vi "Read_Loop.vi"(8 "Status/Errors in":refnum<vi>, 9 "Read bytes parameters in":T1 {"Read bytes"."Max bytes read" format="%#.0f"}, 10 "Timer parameters":refnum<vi>, 11 "Devices":T4) -> (0 "Status/Errors out":refnum<vi>, 1 "Read bytes parameters out":T1 {"Read bytes"."Max bytes read" format="%#.0f"}, 2 "Slave bytes":u8[](array[numeric]), 3 "Master bytes":u8[](array[numeric]), 4 "# Master bytes":u32, 6 "# Slave bytes":u32)   [LabVIEW 2013]
uses:
  Controls/Read_Bytes_Parameters.ctl
  Controls/Stop_Loop.ctl
  Controls/Read_Bytes.ctl
  Controls/Devices.ctl
  Controls/Timer_Elements.ctl
  Controls/Get_Set_Timer_Options.ctl
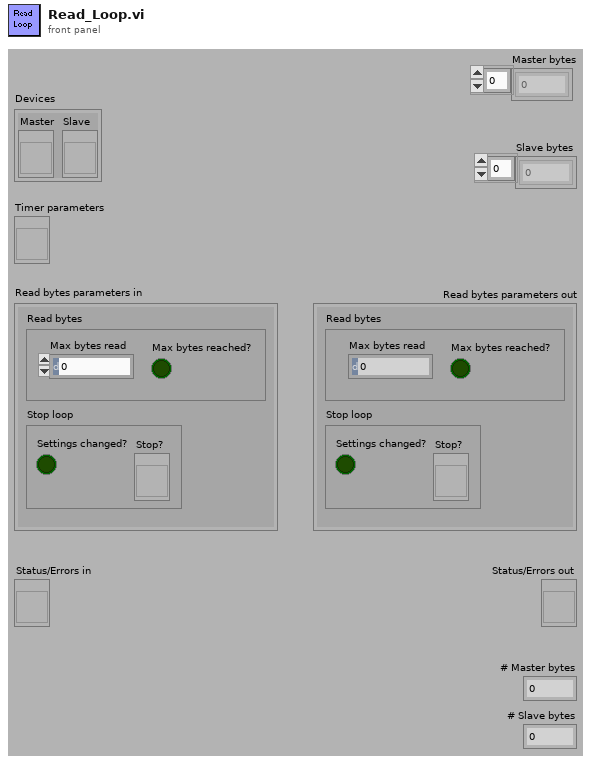
[diagram p1: front panel]
types:
  T1 = typedef "Read_Bytes_Parameters.ctl" = cluster{"Stop loop":T2, "Read bytes":T3}
  T2 = typedef "Stop_Loop.ctl" = cluster{"Settings changed?":bool, "Stop?":refnum<vi>}
  T3 = typedef "Read_Bytes.ctl" = cluster{"Max bytes read":u32, "Max bytes reached?":bool}
  T4 = typedef "Devices.ctl" = cluster{"Master":refnum<vi>, "Slave":refnum<vi>}
  T5 = typedef "Semaphore RefNum" = refnum<k1>
  T6 = typedef "Get_Set_Timer_Options.ctl" = enum16{"Get", "Get cluster", "Set", "Set to current time"}
  T7 = typedef "Timer_Elements.ctl" = enum16{"Default", "Current time", "Time screen updated", "Time controls locked", "Time last device check", "Time last data MAS", "Time last data SLV", "Time bad status MAS", "Time bad status SLV", "Time clock error updated", "Time delay screen update", "Time delay controls", "Time delay device check", "Time until MAS status bad", "Time until SLV status bad", "Time until MAS connection bad", "Time until SLV connection bad", "Time delay clock error update"}
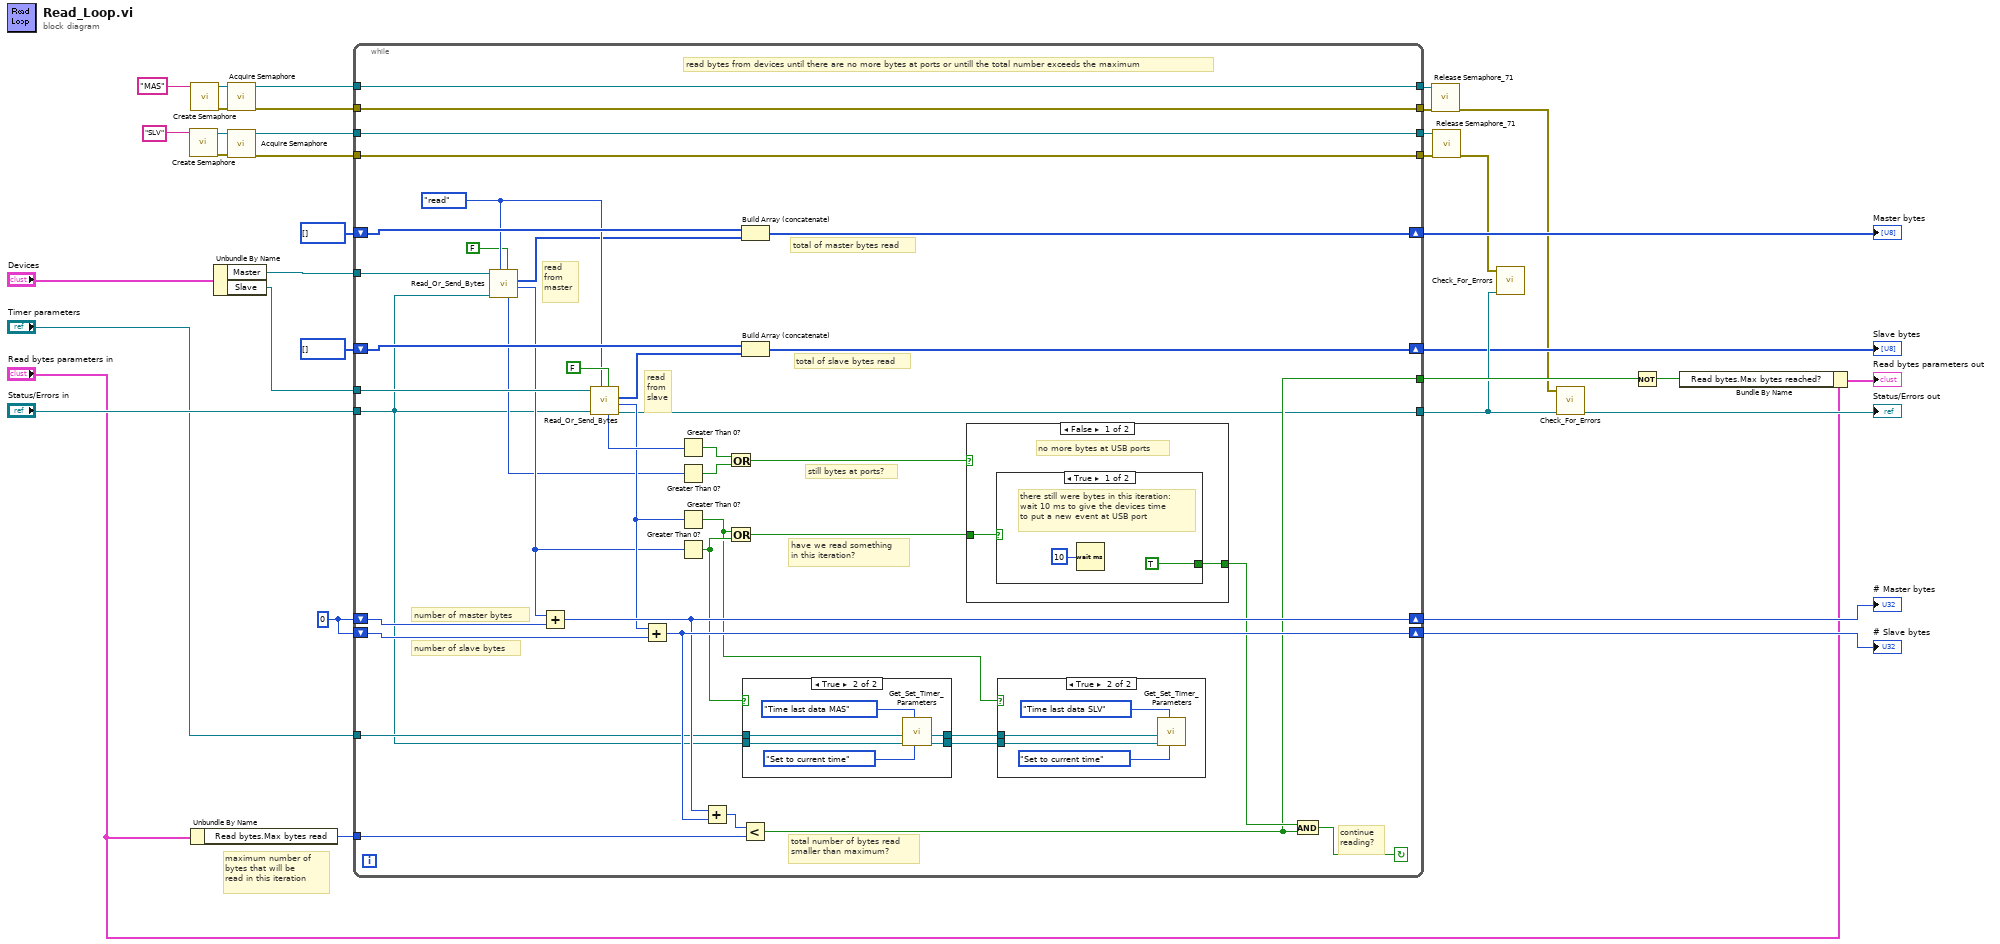
[diagram p0: block diagram]
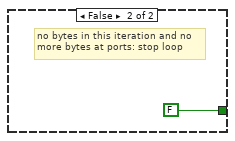
[diagram p4: hidden frame]
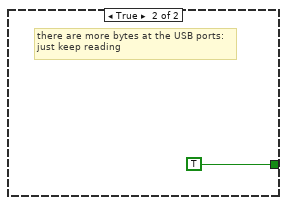
[diagram p5: hidden frame]
diagram:
  w33 = u32 0
  # "maximum number of\nbytes that will be\nread in this iteration"
  n1 = call <vilib>:"Create Semaphore.vi"("name (unnamed)"="SLV") -> ("error out"=w11:errorcluster, "semaphore"=w12:T5)  [unwired: 2 in, 3 out]
  n2 = call <vilib>:"Create Semaphore.vi"("name (unnamed)"="MAS") -> ("error out"=w7:errorcluster, "semaphore"=w8:T5)  [unwired: 2 in, 3 out]
  n3 = Unbundle By Name("Read bytes parameters in") -> ("Read bytes.Max bytes read"=w13:u32)
  n4 = Unbundle By Name("Devices") -> ("Master"=w35:refnum<vi>, "Slave"=w34:refnum<vi>)
  n5 = call <vilib>:"Acquire Semaphore.vi"("error in (no error)"=w7, "semaphore"=w8) -> ("error out"=w24:errorcluster, "semaphore out"=w25:T5)  [unwired: 1 in, 3 out]
  n6 = call <vilib>:"Acquire Semaphore.vi"("error in (no error)"=w11, "semaphore"=w12) -> ("error out"=w21:errorcluster, "semaphore out"=w22:T5)  [unwired: 1 in, 3 out]
  n7 = while {
    tunnel: "Status/Errors in" -> [w36]
    shift-right: [w69] -> w30
    shift-left: w33 -> [w72]
    tunnel: w13 -> [w74]
    shift-right: [w56] -> w17
    shift-left: u8[] [] -> [w57]
    shift-right: [w55] -> w16
    shift-left: u8[] [] -> [w54]
    shift-right: [w70] -> w29
    shift-left: w33 -> [w71]
    tunnel: w35 -> [w42]
    tunnel: w34 -> [w48]
    tunnel: [w43] -> w20
    tunnel: [w62] -> w28
    tunnel: w25 -> [w60]
    tunnel: w24 -> [w61]
    tunnel: [w61] -> w5
    tunnel: [w60] -> w4
    tunnel: w22 -> [w58]
    tunnel: w21 -> [w59]
    tunnel: [w59] -> w2
    tunnel: [w58] -> w1
    tunnel: "Timer parameters" -> [w53]
    stop <- w73 continue-if-true
    w41 = enum8{"read", "write"}."read" ("Read or write?")
    # "have we read something\nin this iteration?"
    # "number of slave bytes"
    # "number of master bytes"
    # "read\nfrom\nmaster"
    # "read\nfrom\nslave"
    # "read bytes from devices until there are no more bytes at ports or untill the total number exceeds the maximum"
    # "total of slave bytes read"
    # "total of master bytes read"
    # "continue\nreading?"
    # "total number of bytes read\nsmaller than maximum?"
    # "still bytes at ports?"
    n8 = call "Read_Or_Send_Bytes.vi"("Aquire semaphore? (t)"=FALSE, "Read or write?"=w41, "Status/Errors in"=w36, "Device in"=w42) -> ("Return count"=w38:u32, "Read buffer"=w39:u8[], "Bytes at Port"=w37:u32)  [unwired: 1 in, 4 out]
    n9 = Add(x=w38, y=w72) -> (x+y=w69:u32)
    n10 = call "Read_Or_Send_Bytes.vi"("Aquire semaphore? (t)"=FALSE, "Read or write?"=w41, "Status/Errors in"=w36, "Device in"=w48) -> ("Status/Errors out"=w43:refnum<vi>, "Return count"=w44:u32, "Read buffer"=w45:u8[], "Bytes at Port"=w46:u32)  [unwired: 1 in, 3 out]
    n11 = Add(x=w44, y=w71) -> (x+y=w70:u32)
    n12 = Greater Than 0?(x=w46) -> (x > 0?=w66:bool)
    n13 = Greater Than 0?(x=w37) -> (x > 0?=w65:bool)
    n14 = Greater Than 0?(x=w44) -> (x > 0?=w49:bool)
    n15 = Greater Than 0?(x=w38) -> (x > 0?=w50:bool)
    n16 = Add(x=w69, y=w70) -> (x+y=w68:u32)
    n17 = Or(x=w66, y=w65) -> (x .or. y?=w64:bool)
    n18 = Or(x=w49, y=w50) -> (x .or. y?=w63:bool)
    n19 = Less?(x=w68, y=w74) -> (x < y?=w62:bool)
    n20 = Build Array (concatenate)(w57, w39) -> (w56:u8[])
    n21 = Build Array (concatenate)(w54, w45) -> (w55:u8[])
    n22 = case shown="True" w50 {
      tunnel: w36 -> [w79 w84]
      tunnel: w53 -> [w80 w83]
      tunnel: [w80 w82] -> w52
      tunnel: [w79 w81] -> w51
      frame False {
      }
      frame True {
        n23 = call "Get_Set_Timer_Parameters.vi"("Get/Set"=Get_Set_Timer_Options."Set to current time", "Element"=Timer_Elements."Time last data MAS", "Status/Errors in"=w84, "Timer parameters in"=w83) -> ("Status/Errors out"=w81:refnum<vi>, "Timer parameters out"=w82:refnum<vi>)  [unwired: 2 in, 4 out]
      }
    }
    n24 = case shown="False" w64 {
      tunnel: w63 -> [w88 _]
      tunnel: [w87 TRUE] -> w67
      frame False {
        # "no more bytes at USB ports"
        n25 = case shown="True" w88 {
          tunnel: [TRUE FALSE] -> w87
          frame True {
            # "there still were bytes in this iteration:\nwait 10 ms to give the devices time\nto put a new event at USB port"
            n26 = Wait (ms)(milliseconds to wait=u32 10) -> ()  [unwired: 1 out]
          }
          frame False {
            # "no bytes in this iteration and no\nmore bytes at ports: stop loop"
          }
        }
      }
      frame True {
        # "there are more bytes at the USB ports:\njust keep reading"
      }
    }
    n27 = case shown="True" w49 {
      tunnel: w51 -> [_ w76]
      tunnel: w52 -> [_ w75]
      frame False {
      }
      frame True {
        n28 = call "Get_Set_Timer_Parameters.vi"("Get/Set"=Get_Set_Timer_Options."Set to current time", "Element"=Timer_Elements."Time last data SLV", "Status/Errors in"=w76, "Timer parameters in"=w75) -> ()  [unwired: 2 in, 6 out]
      }
    }
    n29 = And(x=w67, y=w62) -> (x .and. y?=w73:bool)
  }
  "# Master bytes" <- w30
  "# Slave bytes" <- w29
  "Master bytes" <- w17
  "Slave bytes" <- w16
  n30 = call <vilib>:"Release Semaphore_71.vi"("error in (no error)"=w5, "semaphore"=w4) -> ("error out"=w6:errorcluster)  [unwired: 5 out]
  n31 = call <vilib>:"Release Semaphore_71.vi"("error in (no error)"=w2, "semaphore"=w1) -> ("error out"=w3:errorcluster)  [unwired: 5 out]
  n32 = call "Check_For_Errors.vi"("Status/Errors in"=w20, "error in"=w3) -> ()  [unwired: 10 out]
  n33 = call "Check_For_Errors.vi"("Status/Errors in"=w20, "error in"=w6) -> ("Status/Errors out"=→"Status/Errors out":refnum<vi>)  [unwired: 9 out]
  n34 = Not(x=w28) -> (.not. x?=w26:bool)
  n35 = Bundle By Name(cluster="Read bytes parameters in", "Read bytes.Max bytes reached?"=w26) -> (→"Read bytes parameters out":T1)
